vi "Get Angle.vi"(4 "Axis":T1, 8 "error in (no error)":errorcluster, 11 "instrument.PPMS":refnum<class "instrument.PPMS.lvclass">) -> (0 "error out":errorcluster, 1 "Status":string, 2 "Angle (°)":dbl, 3 "instrument.PPMS out":refnum<class "instrument.PPMS.lvclass">)   [LabVIEW 2019, in "instrument.PPMS.lvclass"]
uses:
  instrument.PPMS.lvclass
  c9205d4d-83b9-4023-b61f-e99dd979e23a.vi
  Typedefs/PPMS.Commands-enum.ctl
  C:/Program Files (x86)/National Instruments/LabVIEW 2019/user.lib/LevyLab/Levylab Instruments/Instrument Types/Cryostat/Instrument.Cryostat.lvclass
  C:/Program Files (x86)/National Instruments/LabVIEW 2019/user.lib/LevyLab/Levylab Instruments/SMOs/Instrument/Instrument.lvclass
  C:/Program Files (x86)/National Instruments/LabVIEW 2019/vi.lib/JKI/JKI SMO/SMO/SMO.lvclass
  <userlib>/LevyLab/Levylab Instruments/Instrument Types/Cryostat/Typedefs/Rotator Axis--Enum.ctl
  <userlib>/LevyLab/Levylab Instruments/Instrument Types/Cryostat/Instrument.Cryostat.lvclass
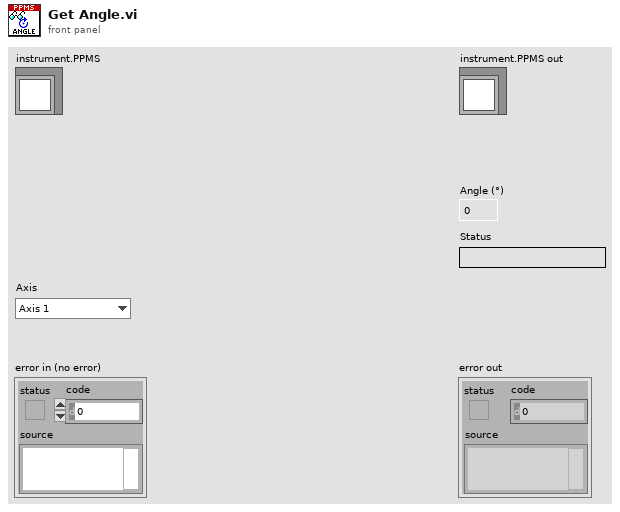
[diagram p1: front panel]
types:
  T1 = typedef "Instrument.Cryostat.lvclass/Rotator Axis--Enum.ctl" = enum16{"Axis 1", "Axis 2"}
  T2 = typedef "instrument.PPMS.lvclass/PPMS.Commands-enum.ctl" = enum16{"Get Angle", "Get Helium Level", "Get Magnet", "Get Temperature", "Set Angle", "Set Chamber", "Set Magnet", "Set Temperature", "getAll"}
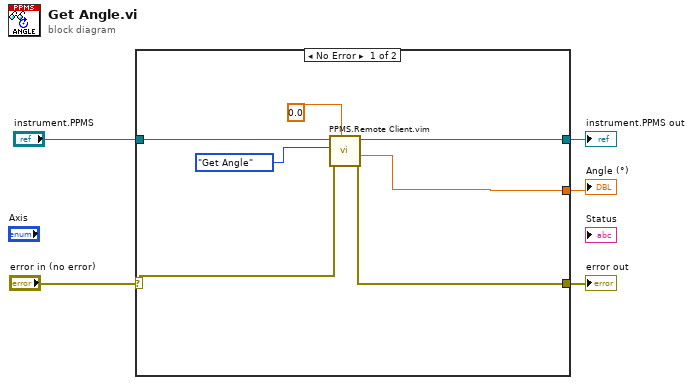
[diagram p0: block diagram]
diagram:
  n1 = case shown="No Error" "error in (no error)" {
    selector: "error in (no error)" -> [w9 w14]
    tunnel: [w6 _] -> w5
    tunnel: [w8 w14] -> w4
    tunnel: "instrument.PPMS" -> [w12 w13]
    tunnel: [w11 w13] -> w1
    frame No Error {
      n2 = call "PPMS.Remote Client.vim"("Data Out type"=0.0, "error in (no error)"=w9, "Command"=PPMS.Commands-enum."Get Angle", "instrument.PPMS in"=w12) -> ("error out"=w8:errorcluster, "Data out"=w6:dbl, "instrument.PPMS out"=w11:refnum<class "instrument.PPMS.lvclass">)  [unwired: 5 in]
    }
    frame Error {
    }
  }
  "error out" <- w4
  "instrument.PPMS out" <- w1
  "Angle (°)" <- w5
